vi "PS90_TargetEx.vi"(5 "read?":bool, 7 "Control unit ID":i32=1 min=1 max=10, 8 "error in (no error)":errorcluster, 9 "dValue-In":dbl format="%.4f", 10 "Axis number":i32=1 min=1 max=9, 11 "DLOwis.lvclass":refnum<class "DLOwis.lvclass">) -> (0 "error out":errorcluster, 1 "dValue-Out":dbl format="%.4f", 3 "DLOwis.lvclass":refnum<class "DLOwis.lvclass">)   [LabVIEW 2018, in "DLOwis.lvclass"]
doc: "PS90_TargetEx.vi, created: 13.11.2006 alex; last change: 21.07.2016 alex;\n\n<B>FUNCTIONS:</B> \n\n<B>Read:</B> FALSE: read target position or distance \nof an axis (values in selected unit).\n<B>Write:</B> TRUE: set target position or distance \nof an axis (values in selected unit).\nThe definition depends on the target mode. The sign determines\nthe positioning direction.\n----------------------------------------------------------------------------------------\n<B>INPUT:</B>\n[TF] <B>function:</B> function selector. (Read, Write)\n[I32] <B>Control unit ID:</B> control unit index. (Default=1, Range=1...10)\n[I32] <B>Axis number:</B> axis number. (Default=1, Range=1...9)\n[DBL] <B>dValue-In:</B> target position or distance. (only for Write: Default=0.0)\n[CLU] <B>error in</B>\n----------------------------------------------------------------------------------------\n<B>OUTPUT:</B>\n[DBL] <B>dValue-Out:</B> target position or distance. (for Write: dValue-Out=dValue-In)\n[CLU] <B>error out</B>\n----------------------------------------------------------------------------------------\n<B>SUB-VIs:</B>\nPS90_GetReadError.vi\n----------------------------------------------------------------------------------------\n<B>EXT-Calls:</B>\nps90.dll (V2.00)\n----------------------------------------------------------------------------------------"
uses:
  DLOwis.lvclass
  C:/Users/Sergey Denisov/Documents/REPS/TRANCON/Classes/Delay Line/DelayLine.lvclass
  DelayLine.lvclass/DelayLine.ctl
  DelayLine.lvclass
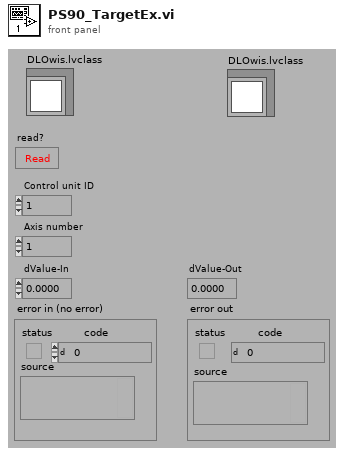
[diagram p1: front panel]
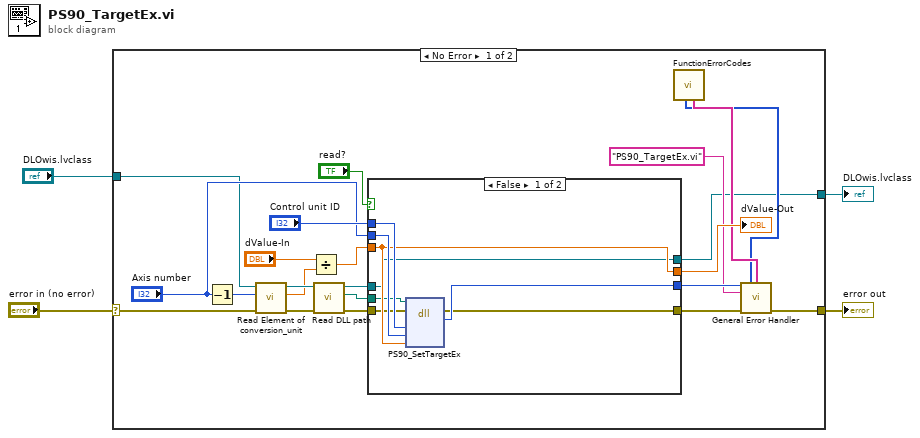
[diagram p0: block diagram]
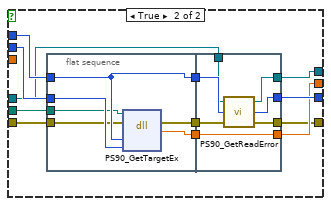
[diagram p2: hidden frame]
diagram:
  n1 = case shown="No Error" "error in (no error)" {
    selector: "error in (no error)" -> [w11 w60]
    tunnel: [w26 w60] -> w4
    tunnel: "DLOwis.lvclass" -> [w6 w61]
    tunnel: [w16 w61] -> w2
    frame No Error {
      n2 = Decrement(x="Axis number") -> (x-1=w5:i32)
      n3 = call "Read Element of conversion_unit.vi"("error in (no error)"=w11, "axis"=w5, "DLOwis in"=w6) -> ("error out"=w10:errorcluster, "Numeric"=w8:dbl, "DLOwis out"=w9:refnum<class "DLOwis.lvclass">)  [unwired: 6 in]
      n4 = Divide(x="dValue-In", y=w8) -> (x/y=w13:dbl)
      n5 = call "Read DLL path.vi"("error in (no error)"=w10, "DelayLine in"=w9) -> ("error out"=w17:errorcluster, "DLL path"=w14:path, "DelayLine out"=w18:refnum<class "DLOwis.lvclass">)  [unwired: 7 in]
      n6 = case shown="False" "read?" {
        tunnel: "Control unit ID" -> [w33 w45]
        tunnel: [w34 w46] -> w23
        tunnel: w13 -> [w31 _]
        tunnel: [w31 w44] -> w22
        tunnel: "Axis number" -> [w32 w43]
        tunnel: w18 -> [w28 w40]
        tunnel: w17 -> [w30 w39]
        tunnel: [w28 w37] -> w16
        tunnel: [w29 w36] -> w15
        tunnel: w14 -> [w27 w35]
        frame False {
          n7 = dll-call lib="C:/Users/Sergey Denisov/Documents/REPS/TRANCON/DLL/ps90.dll" fn="PS90_SetTargetEx" label="PS90_Set\nTargetEx"(path in=w27, error in=w30, "Index"=w33, "AxisNr"=w32, "dValue"=w31) -> (error out=w29:errorcluster, "Rückgabetyp"=w34:i32)  [unwired: 4 in, 1 out]
        }
        frame True {
          n8 = flat-sequence {
            tunnel: w45 -> [w52]
            tunnel: [w52] -> w42
            tunnel: [w51] -> w41
            tunnel: w43 -> [w50]
            tunnel: w39 -> [w49]
            tunnel: [w48] -> w38
            tunnel: w35 -> [w47]
            tunnel: [w59] -> w46
            tunnel: w42 -> [w58]
            tunnel: [w57] -> w44
            tunnel: w41 -> [w57]
            tunnel: w40 -> [w56]
            tunnel: w38 -> [w55]
            tunnel: [w54] -> w37
            tunnel: [w53] -> w36
            frame #0 {
              n9 = dll-call lib="C:/Users/Sergey Denisov/Documents/REPS/TRANCON/DLL/ps90.dll" fn="PS90_GetTargetEx" label="PS90_Get\nTargetEx"(path in=w47, error in=w49, "Index"=w52, "AxisNr"=w50) -> (error out=w48:errorcluster, "Rückgabetyp"=w51:dbl)  [unwired: 3 in, 1 out]
            }
            frame #1 {
              n10 = call "PS90_GetReadError.vi"("error in (no error)"=w55, "Control unit ID"=w58, "DLOwis.lvclass"=w56) -> ("error IO"=w53:errorcluster, "Read error"=w59:i32, "DLOwis.lvclass"=w54:refnum<class "DLOwis.lvclass">)
            }
          }
        }
      }
      "dValue-Out" <- w22
      n11 = call "FunctionErrorCodes.vi"() -> ("[user-defined codes]"=w19:i32[], "[user-defined descriptions]"=w20:string[])  [unwired: 8 in]
      n12 = call <vilib>:"General Error Handler.vi"("[error code] (0)"=w23, "[user-defined codes]"=w19, "[user-defined descriptions]"=w20, "[error source] (\" \")"="PS90_TargetEx.vi" ("[error source] (\" \")"), "error in (no error)"=w15) -> ("error out"=w26:errorcluster)  [unwired: 6 in, 4 out]
    }
    frame Error {
    }
  }
  "error out" <- w4
  "DLOwis.lvclass" <- w2
